vi "盐度计算.vi"(10 "spCond":dbl, 11 "Temp":dbl) -> (2 "saltresult":dbl, 3 "cond":dbl)   [LabVIEW 2016, in "斯坦道多参数.lvlib"]
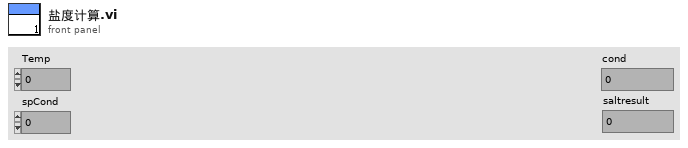
[diagram p1: front panel]
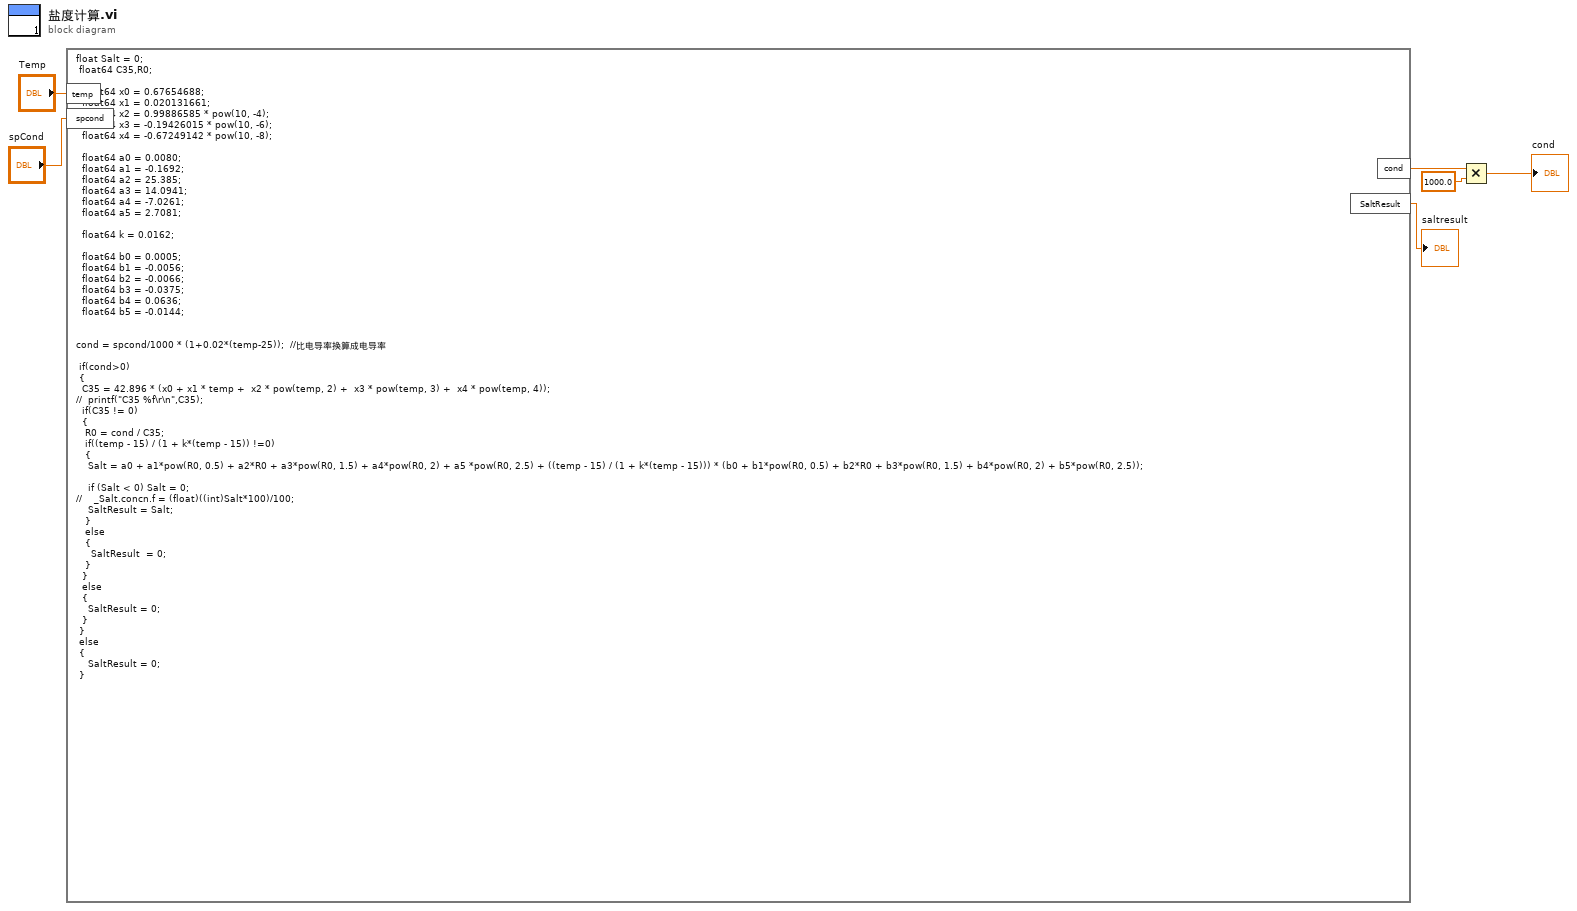
[diagram p0: block diagram]
diagram:
  n1 = formula code="float Salt = 0;\n\tfloat64 C35,R0;\n\n\t\tfloat64 x0 = 0.67654688;\n\t\tfloat64 x1 = 0.020131661;\n\t\tfloat64 x2 = 0.99886585 * pow(10, -4);\n\t\tfloat64 x3 = -0.19426015 * pow(10, -6);\n\t\tfloat64 x4 = -0.67249142 * pow(10, -8);\n\n\t\tfloat64 a0 = 0.0080;\n\t\tfloat64 a1 = -0.1692;\n\t\tfloat64 a2 = 25.385;\n\t\tfloat64 a3 = 14.0941;\n\t\tfloat64 a4 = -7.0261;\n\t\tfloat64 a5 = 2.7081;\n\n\t\tfloat64 k = 0.0162;\n\n\t\tfloat64 b0 = 0.0005;\n\t\tfloat64 b1 = -0.0056;\n\t\tfloat64 b2 = -0.0066;\n\t\tfloat64 b3 = -0.0375;\n\t\tfloat64 b4 = 0.0636;\n\t\tfloat64 b5 = -0.0144;\n\n\ncond = spcond/1000 * (1+0.02*(temp-25));  //比电导率换算成电导率\n\n\tif(cond>0)\n\t{\n\t\tC35 = 42.896 * (x0 + x1 * temp +  x2 * pow(temp, 2) +  x3 * pow(temp, 3) +  x4 * pow(temp, 4));   \n//\t\tprintf(\"C35 %f\\r\\n\",C35);  \n\t\tif(C35 != 0)\n\t\t{\n\t\t\tR0 = cond / C35;\n\t\t\tif((temp - 15) / (1 + k*(temp - 15)) !=0)\n\t\t\t{\n\t\t\t\tSalt = a0 + a1*pow(R0, 0.5) + a2*R0 + a3*pow(R0, 1.5) + a4*pow(R0, 2) + a5 *pow(R0, 2.5) + ((temp - 15) / (1 + k*(temp - 15))) * (b0 + b1*pow(R0, 0.5) + b2*R0 + b3*pow(R0, 1.5) + b4*pow(R0, 2) + b5*pow(R0, 2.5));\n\t\t\t   \t \n\t\t\t\tif (Salt < 0)\tSalt = 0; \n//\t\t\t\t_Salt.concn.f = (float)((int)Salt*100)/100;\n\t\t\t\tSaltResult = Salt;\n\t\t\t}\n\t\t\telse\n\t\t\t{\n\t\t\t\t\tSaltResult  = 0;\n\t\t\t}\n\t\t}\n\t\telse\n\t\t{\n\t\t\t\tSaltResult = 0;\n\t\t}\n\t}\n\telse\n\t{\n\t\t\t\tSaltResult = 0;\n\t}"("temp"="Temp", "spcond"="spCond") -> ("SaltResult"=→"saltresult":dbl, "cond"=w3:dbl)
  n2 = Multiply(x=w3, y=1000.0) -> (x*y=→"cond":dbl)
